vi "ModFractionPoly.vi"   [LabVIEW 2022 SP3]
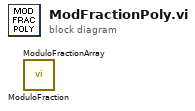
[diagram p0: block diagram]
diagram:
  n1 = call "ModuloFraction.vi"() -> ()  [unwired: 3 in, 1 out]
  n2 = call "ModuloFractionArray.vi"() -> ()  [unwired: 3 in, 1 out]
